vi "Read Key BOOL.vi"(7 "Section Name":string, 8 "error in":errorcluster, 9 "Default Value":bool, 10 "Key Name":string, 11 "Config Cluster in":T1) -> (0 "error out":errorcluster, 1 "Value":bool, 2 "Found?":bool, 3 "Config Cluster out":T1)   [LabVIEW 2017]
uses:
  Config Cluster.ctl
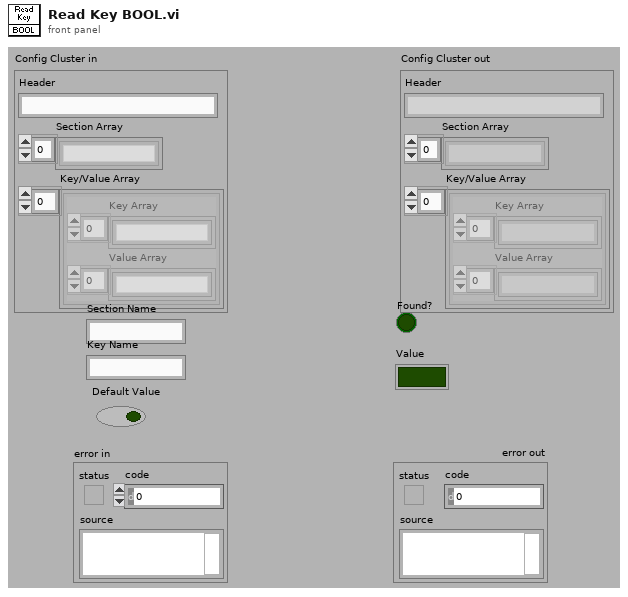
[diagram p1: front panel]
types:
  T1 = typedef "Config Cluster.ctl" = cluster{"Header":string, "Section Array":string[], "Key/Value Array":cluster{"Key Array":string[], "Value Array":string[]}[]}
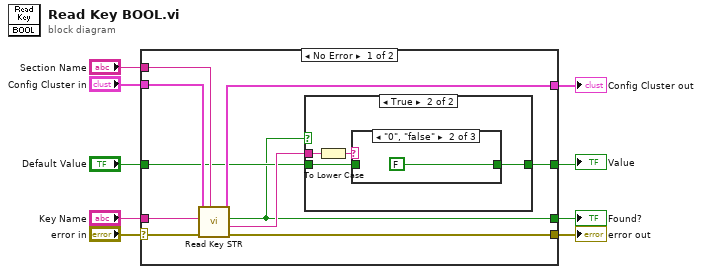
[diagram p0: block diagram]
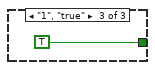
[diagram p4: hidden frame]
diagram:
  n1 = case shown="No Error" "error in" {
    selector: "error in" -> [w18 w29]
    tunnel: [w10 w29] -> w8
    tunnel: "Config Cluster in" -> [w17 w30]
    tunnel: [w16 w30] -> w6
    tunnel: "Section Name" -> [w19 _]
    tunnel: "Key Name" -> [w15 _]
    tunnel: [w12 w28] -> w3
    tunnel: "Default Value" -> [w13 w28]
    tunnel: [w11 _] -> w1
    frame No Error {
      n2 = call "Read Key STR.vi"("Section Name"=w19, "error in"=w18, "Key Name"=w15, "Config Cluster in"=w17) -> ("error out"=w10:errorcluster, "Value"=w14:string, "Found?"=w11:bool, "Config Cluster out"=w16:T1)  [unwired: 4 in]
      n3 = case shown="True" w11 {
        tunnel: w14 -> [_ w23]
        tunnel: [w20 w22] -> w12
        tunnel: w13 -> [w20 w21]
        frame False {
        }
        frame True {
          n4 = To Lower Case(string=w23) -> (all lower case string=w24:string)
          n5 = case shown="\"0\", \"false\"" w24 {
            tunnel: w21 -> [w25 _ _]
            tunnel: [w25 FALSE TRUE] -> w22
            frame Default {
            }
            frame "0", "false" {
            }
            frame "1", "true" {
            }
          }
        }
      }
    }
    frame Error {
    }
  }
  "error out" <- w8
  "Config Cluster out" <- w6
  "Value" <- w3
  "Found?" <- w1
